vi "IR test 001.vi"() -> ()   [LabVIEW 2019]
uses:
  low level/IR sensor/IR sensor.lvclass
  <vilib>/Platform/TimedLoop/XDataNode/timing_clust.ctl
  <vilib>/Platform/TimedLoop/XDataNode/nitl_modes.ctl
  <vilib>/Platform/TimedLoop/XDataNode/wakeup.ctl
  <vilib>/platform/TimedLoop/XDataNode/XDataNode.xnode
  <vilib>/Platform/TimedLoop/XDataNode/XDNodeRunTimeDep.lvlib
panel:
  in  "stop":bool
  out "error out":errorcluster
  out "IR sensor out":refnum<class "IR sensor.lvclass">
  out "IR":u16
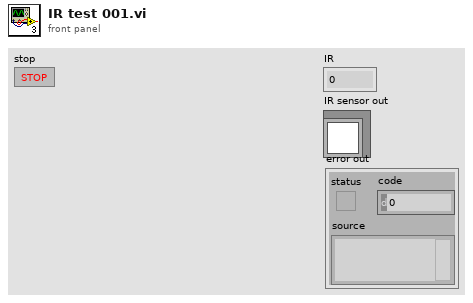
[diagram p1: front panel]
types:
  T1 = enum16{"IR.1", "IR.2", "IR.3", "IR.4", "IR.5", "IR.6", "IR.7", "IR.8"}
  T2 = typedef "XDNodeRunTimeDep.lvlib/timing_clust.ctl" = cluster{"Expected End [f-1]":u64, "Actual End [f-1]":u64, "Finished Late? [f-1]":bool, "Expected End [i-1]":u64, "Actual End [i-1]":u64, "Finished Late? [i-1]":bool, "Expected Start [i]":u64, "Actual Start [i]":u64, "Expected Start [f]":u64, "Actual Start [f]":u64, "Source Name":string, "Structure Name":string, "Period":i64, "Deadline":i64, "Offset":i64, "Start":i64, "Priority":i32, "Timeout":i32, "Mode":T3, "Wakeup Reason":T4, "Error":errorcluster, "Source Type":string, "Secondary Source Type":string, "Global End Time":u64, "Global Start Time":u64, "Frame Duration":u64, "Iteration Duration":u64, "Assigned CPU":i32, "I/O Scan Engine Mode":u32}
  T3 = typedef "XDNodeRunTimeDep.lvlib/nitl_modes.ctl" = enum32{"No Change", "Process missed periods, maintain original phase", "Discard missed periods, maintain original phase", "Process missed periods, ignore original phase", "Discard missed periods, ignore original phase"}
  T4 = typedef "XDNodeRunTimeDep.lvlib/wakeup.ctl" = enum32{"Normal", "Aborted", "Asynchronous wakeup", "Timing source error", "Timed loop error", "Timeout"}
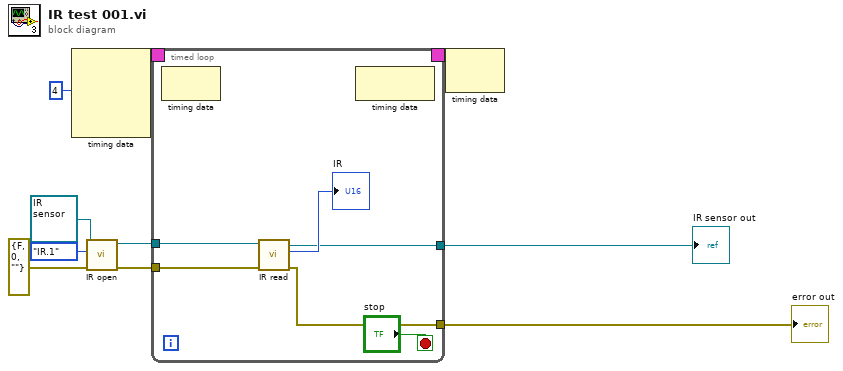
[diagram p0: block diagram]
diagram:
  n1 = node-c288(i64 4 ("Period")) -> (w5:T2)  [unwired: 3 in]
  n2 = call-dynamic "IR open.vi"("error in (no error)"=errorcluster {"status"=FALSE, "code"=0, "source"=""}, "IR pin"=T1."IR.1", "IR sensor in"=refnum<class "IR sensor.lvclass"> refnum) -> ("error out"=w9:errorcluster, "IR sensor out"=w10:refnum<class "IR sensor.lvclass">)  [unwired: 7 in]
  n3 = timed-loop {
    timing: w5 -> [_]
    timing-out: [_] -> w4
    tunnel: w10 -> [w16]
    tunnel: w9 -> [w15]
    tunnel: [w13] -> w2
    tunnel: [w12] -> w1
    stop <- "stop" stop-if-true
    n4 = node-c288() -> ()  [unwired: 1 in, 1 out]
    n5 = call-dynamic "IR read.vi"("error in (no error)"=w15, "IR sensor in"=w16) -> ("error out"=w12:errorcluster, "IR"=→"IR":u16, "IR sensor out"=w13:refnum<class "IR sensor.lvclass">)  [unwired: 7 in]
    n6 = node-c288() -> ()  [unwired: 1 in, 1 out]
  }
  "IR sensor out" <- w2
  "error out" <- w1
  n7 = node-c288(w4) -> ()  [unwired: 1 out]
